vi "SubVI_IntakeReadEncoder_TeleOp.vi"() -> ()   [LabVIEW 2017]
panel:
  out "Waveform Chart":cluster{"Distance":dbl, "current (A)":dbl}(graph)
  out "EncoderCurrent":dbl
  out "Stopped":bool
  out "EncoderRate":dbl
  out "EncoderDistance":dbl
  out "EncoderDirection":bool
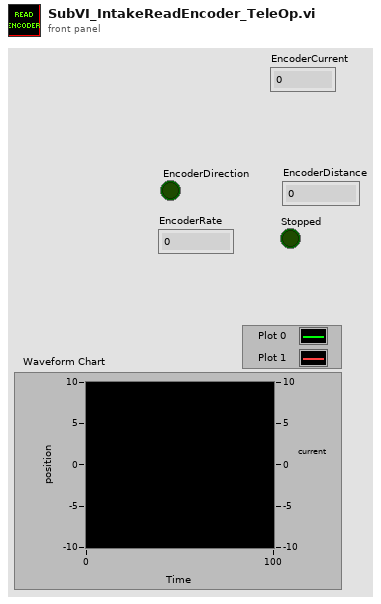
[diagram p1: front panel]
types:
  T1 = typedef "WPI_EncoderDevRef.ctl" = cluster{"DevStatus":errorcluster, "EncoderIndex":T2, "CounterIndex":T3, "DistancePerCount":dbl, "Decoding Type":T4}
  T2 = typedef "FPGA_EncoderIdx.ctl" = enum8{"Enc 0", "Enc 1", "Enc 2", "Enc 3", "Enc 4", "Enc 5", "Enc 6", "Enc 7", "Invalid"}
  T3 = typedef "FPGA_CounterCtrSystemIndex.ctl" = enum8{"Ctr 0", "Ctr 1", "Ctr 2", "Ctr 3", "Ctr 4", "Ctr 5", "Ctr 6", "Ctr 7", "Invalid"}
  T4 = typedef "WPI_EncoderType.ctl" = enum16{"1x", "2x", "4x"}
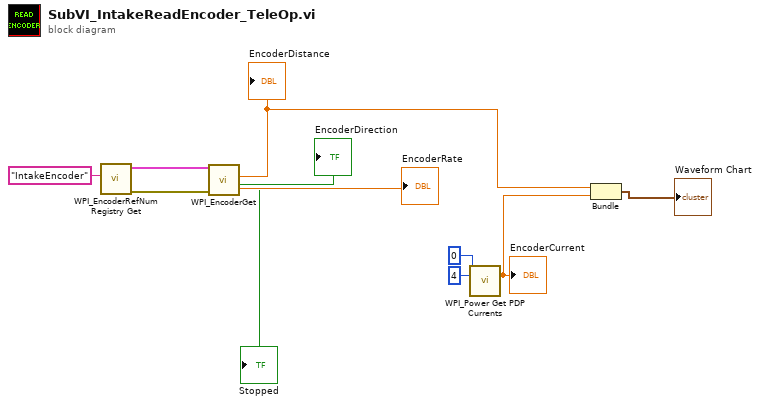
[diagram p0: block diagram]
diagram:
  n1 = call <vilib>:"WPI_EncoderRefNum Registry Get.vi"("refnum name"="IntakeEncoder") -> ("error out"=w9:errorcluster, "EncoderDevRef"=w10:T1)  [unwired: 9 in]
  n2 = call <vilib>:"WPI_EncoderGet.vi"("error in (no error)"=w9, "EncoderDevRef"=w10) -> ("Direction"=→"EncoderDirection":bool, "Distance"=w5:dbl, "Rate"=→"EncoderRate":dbl, "Stopped"=→"Stopped":bool)  [unwired: 4 in, 2 out]
  "EncoderDistance" <- w5
  n3 = call <vilib>:"WPI_Power Get PDP Currents.vi"("Power Distribution Panel (0)"=u8 0, "PDP Channel"=4) -> ("current (A)"=w2:dbl)  [unwired: 11 in, 2 out]
  "EncoderCurrent" <- w2
  n4 = Bundle("Distance"=w5, "current (A)"=w2) -> (→"Waveform Chart":cluster{"Distance":dbl, "current (A)":dbl})  [unwired: 1 in]
